vi "Multicast Endpoint.vi"(8 "error in (no error)":errorcluster, 11 "Group in":refnum<class "Group Config.lvclass">) -> (0 "error out":errorcluster, 2 "Multicast Endpoint":T1, 3 "Group out":refnum<class "Group Config.lvclass">)   [LabVIEW 2020, in "VolatusConfig.lvlib" / "Group Config.lvclass"]
uses:
  Group Config.lvclass
  C:/dev/lv20CE/relink/lv-volatus/VolatusConfig/VolatusConfigElement/VolatusConfigElement.lvclass
  lv-vecto/VectoConfig/Endpoint.ctl
  VolatusConfigElement/VolatusConfigElement.lvclass/VolatusConfigElement.ctl
  Group Config.lvclass/Group Config.ctl
  lv-cdm/CDM-Config/Config Element/Config Element.lvclass
  VolatusConfigElement/VolatusConfigElement.lvclass
  lv-vecto/VectoConfig/VectoConfig.lvlib
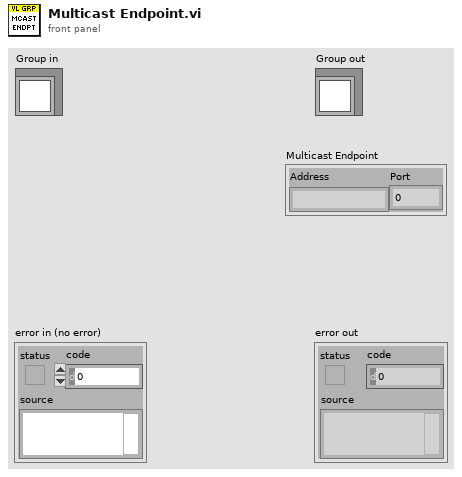
[diagram p1: front panel]
types:
  T1 = typedef "VectoConfig.lvlib/Endpoint.ctl" = cluster{"Address":string, "Port":u16}
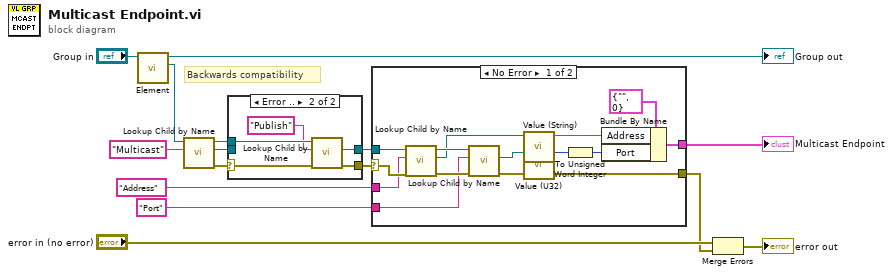
[diagram p0: block diagram]
diagram:
  # "Backwards compatibility"
  n1 = call "Element.vi"("VolatusConfigElement in"="Group in") -> ("Element"=w6:refnum<class "Config Element.lvclass">, "VolatusConfigElement out"=→"Group out":refnum<class "Group Config.lvclass">)  [unwired: 9 in]
  n2 = call "Lookup Child by Name.vi"("Name"="Multicast", "Config Element in"=w6) -> ("error out"=w5:errorcluster, "Child"=w3:refnum<class "Config Element.lvclass">, "Config Element out"=w4:refnum<class "Config Element.lvclass">)  [unwired: 6 in, 1 out]
  n3 = case shown="Error .." w5 {
    selector: w5 -> [w16 w21]
    tunnel: w4 -> [_ w22]
    tunnel: w3 -> [w17 _]
    tunnel: [w17 w19] -> w2
    tunnel: [w16 w20] -> w1
    frame No Error {
    }
    frame Error {
      n4 = call "Lookup Child by Name.vi"("error in (no error)"=w21, "Name"="Publish", "Config Element in"=w22) -> ("error out"=w20:errorcluster, "Child"=w19:refnum<class "Config Element.lvclass">)  [unwired: 5 in, 2 out]
    }
  }
  n5 = case shown="No Error" w1 {
    selector: w1 -> [w34 _]
    tunnel: w2 -> [w35 _]
    tunnel: "Address" ("Name") -> [w33 _]
    tunnel: "Port" ("Name") -> [w31 _]
    tunnel: [w24 _] -> w9
    tunnel: [w23 _] -> w8
    frame No Error {
      n6 = call "Lookup Child by Name.vi"("error in (no error)"=w34, "Name"=w33, "Config Element in"=w35) -> ("error out"=w36:errorcluster, "Child"=w25:refnum<class "Config Element.lvclass">, "Config Element out"=w32:refnum<class "Config Element.lvclass">)  [unwired: 5 in, 1 out]
      n7 = call "Lookup Child by Name.vi"("error in (no error)"=w36, "Name"=w31, "Config Element in"=w32) -> ("error out"=w24:errorcluster, "Child"=w29:refnum<class "Config Element.lvclass">)  [unwired: 5 in, 2 out]
      n8 = call "Value (String).vi"("Config Element in"=w25) -> ("String Value"=w26:string)  [unwired: 9 in, 1 out]
      n9 = call "Value (U32).vi"("Config Element in"=w29) -> ("U32 Value"=w28:u32)  [unwired: 9 in, 1 out]
      n10 = To Unsigned Word Integer(number=w28) -> (unsigned 16bit integer=w27:u16)
      n11 = Bundle By Name(cluster=T1 {"Address"="", "Port"=0} ("Endpoint"), "Address"=w26, "Port"=w27) -> (w23:T1)
    }
    frame Error {
      # "Doesn't have publish config which is fine, it just won't be published."
    }
  }
  "Multicast Endpoint" <- w8
  n12 = Merge Errors("error in (no error)", w9) -> (→"error out":errorcluster)
